vi "Action.vi"(8 "error in (no error)":errorcluster, 10 "OOQMH in":refnum<class "OOQMH.lvclass">, 11 "Set Loop Period in":refnum<class "Set Loop Period.lvclass">) -> (0 "error out":errorcluster, 2 "OOQMH out":refnum<class "OOQMH.lvclass">, 3 "Set Loop Period out":refnum<class "Set Loop Period.lvclass">)   [LabVIEW 2024, in "PID Loop.lvlib" / "Set Loop Period.lvclass"]
uses:
  OOQMH/OOQMH/OOQMH.lvclass
  Set Loop Period.lvclass
  Set Loop Period.lvclass/Set Loop Period.ctl
  PID Loop/PID Loop.lvclass
  C:/Users/uspoaotto/OneDrive - Oregon Tool/Desktop/working copies/helperLoop/src/OOQMH/OOQMH/OOQMH.lvclass
  C:/Users/uspoaotto/OneDrive - Oregon Tool/Desktop/working copies/helperLoop/src/PID Loop/PID Loop/PID Loop.lvclass
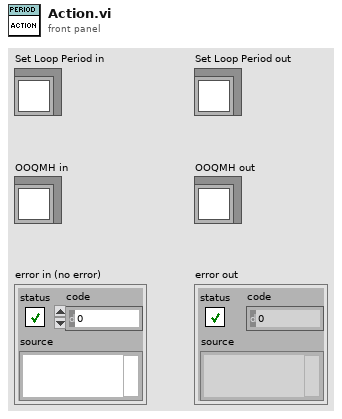
[diagram p1: front panel]
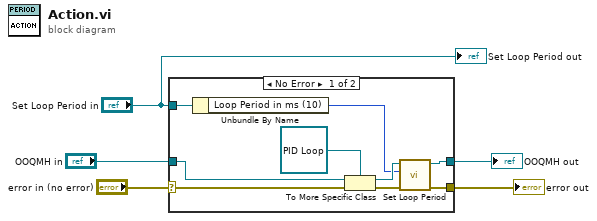
[diagram p0: block diagram]
diagram:
  n1 = case shown="No Error" "error in (no error)" {
    selector: "error in (no error)" -> [w6 w15]
    tunnel: "OOQMH in" -> [w14 w16]
    tunnel: [w11 w16] -> w4
    tunnel: [w10 w15] -> w3
    tunnel: "Set Loop Period in" -> [w8 _]
    frame No Error {
      n2 = Unbundle By Name(w8) -> ("Loop Period in ms (10)"=w7:u32)
      n3 = To More Specific Class(target class=refnum<class "PID Loop.lvclass"> refnum ("PID Loop in"), reference=w14, error in=w6) -> (specific class reference=w13:refnum<class "PID Loop.lvclass">, error out=w12:errorcluster)
      n4 = call-dynamic "Set Loop Period.vi"("error in (no error)"=w12, "Loop Period in ms (10)"=w7, "PID Loop in"=w13) -> ("error out"=w10:errorcluster, "PID Loop out"=w11:refnum<class "PID Loop.lvclass">)  [unwired: 7 in]
    }
    frame Error {
    }
  }
  "error out" <- w3
  "OOQMH out" <- w4
  "Set Loop Period out" <- "Set Loop Period in"
